vi "Transformation Matrix.vi"(9 "Axis":enum16{"x", "y", "z"}(ring), 10 "Angle (degrees)":dbl, 11 "Translation":cluster{"X":dbl, "Y":dbl, "Z":dbl}) -> (3 "Transformation Matrix":T1)   [LabVIEW 2024]
uses:
  <vilib>/Analysis/Matrix/Datatypes/RealMatrix.ctl
  <vilib>/Analysis/baseanly.llb/Real A x B.vi
  <vilib>/Analysis/NI_AALBase.lvlib
  <vilib>/Analysis/Matrix/NI_Matrix.lvlib
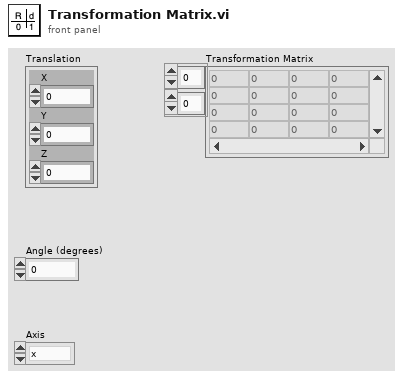
[diagram p1: front panel]
types:
  T1 = typedef "NI_Matrix.lvlib/RealMatrix.ctl" = dbl[][]
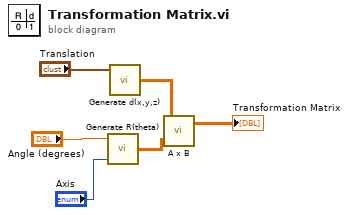
[diagram p0: block diagram]
diagram:
  n1 = call <userlib>:"Generate R(theta).vi"("Axis"="Axis", "Angle (degrees)"="Angle (degrees)") -> ("Transformation Matrix"=w5:T1)  [unwired: 1 in]
  n2 = call <userlib>:"Generate d(x,y,z).vi"("Translation"="Translation") -> ("Transformation Matrix"=w6:T1)  [unwired: 2 in]
  n3 = call-poly <vilib>:"A x B.vi"("B"=w5, "A"=w6) -> ("A x B"=→"Transformation Matrix":T1)  [unwired: 1 out]
